vi "voltage_to_temperature.vi"(8 "error in":errorcluster, 11 "Voltage In":dbl) -> (0 "error out":errorcluster, 3 "Temp Out":dbl)   [LabVIEW 2020]
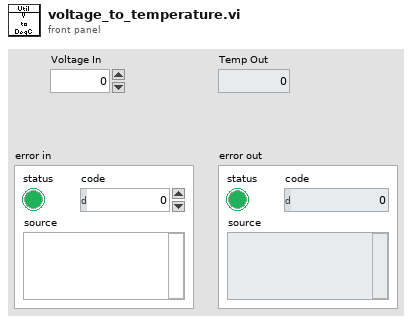
[diagram p1: front panel]
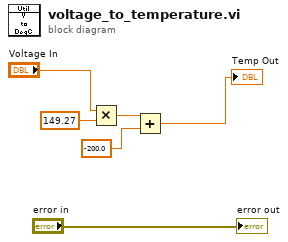
[diagram p0: block diagram]
diagram:
  n1 = Multiply(x="Voltage In", y=149.27) -> (x*y=w3:dbl)
  n2 = Add(x=w3, y=-200.0) -> (x+y=→"Temp Out":dbl)
  "error out" <- "error in"
